vi "Write Instrument Dataset Msg.vi"(10 "Instrument.lvlib:Instrument Dataset Msg.lvclass":refnum<class "Instrument Dataset Msg.lvclass">, 11 "Instrument in":refnum<class "Instrument.lvclass">) -> (3 "Instrument out":refnum<class "Instrument.lvclass">)   [LabVIEW 2019, in "Instrument.lvlib" / "Instrument.lvclass"]
uses:
  Instrument.lvclass
  Instrument Messages/Instrument Dataset Msg/Instrument Dataset Msg.lvclass
  Instrument.lvclass/Instrument.ctl
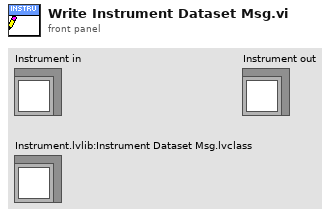
[diagram p1: front panel]
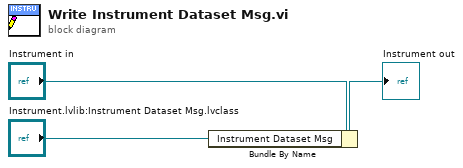
[diagram p0: block diagram]
diagram:
  n1 = Bundle By Name(cluster="Instrument in", "Instrument Dataset Msg"="Instrument.lvlib:Instrument Dataset Msg.lvclass") -> (→"Instrument out":refnum<class "Instrument.lvclass">)
